vi "MyrioProject.vi"() -> ()   [LabVIEW 2018]
doc: "The myRIO Project template acquires acceleration data from the onboard accelerometer and displays the changes of acceleration values in a waveform chart."
uses:
  <vilib>/myRIO/Common/Instrument Driver Framework/Utilities/typedefs/Generic FPGA Reference.ctl
  <vilib>/myRIO/Common/Instrument Driver Framework/Utilities/typedefs/myRIO v1.0 Reference.ctl
  <vilib>/myRIO/Common/Instrument Driver Framework/Utilities/typedefs/Hardware Version Enum.ctl
  <vilib>/myRIO/Common/Instrument Driver Framework/Utilities/typedefs/myRIO Generic Hardware Reference.ctl
  <vilib>/userdefined/High Color/nirio_resource_hc.ctl
  <vilib>/myRIO/Common/Instrument Driver Framework/myRIO v1.0/Encoder/typedefs/Encoder Channels Enum.ctl
  <vilib>/myRIO/Instrument Drivers/Onboard IO/Encoder/typedefs/Encoder Reference.ctl
  <vilib>/myRIO/Instrument Drivers/Onboard IO/Encoder/Encoder.lvlib
  <vilib>/myRIO/Common/Instrument Driver Framework/myRIO v1.0/Encoder/typedefs/Encoder Signal Mode.ctl
  <vilib>/myRIO/Instrument Drivers/Onboard IO/Encoder/vis/myRIO Encoder Open.xnode
  <vilib>/myRIO/Common/Instrument Driver Framework/myRIO v1.0/Encoder/vis/myRIO v1.1 Open Encoder.vi
  <vilib>/myRIO/Common/Instrument Driver Framework/myRIO v1.0/Encoder/vis/myRIO v1.0 Configure Encoder.vi
  <vilib>/myRIO/Common/Instrument Driver Framework/myRIO v1.0/Encoder/typedefs/Encoder Configuration v1.0.ctl
  <vilib>/myRIO/Instrument Drivers/Onboard IO/PWM/typedefs/PWM Configuration.ctl
  <vilib>/myRIO/Instrument Drivers/Onboard IO/PWM/PWM.lvlib
  <vilib>/myRIO/Common/Instrument Driver Framework/myRIO v1.0/PWM/typedefs/PWM Channels Enum.ctl
  <vilib>/myRIO/Instrument Drivers/Onboard IO/PWM/typedefs/PWM Reference.ctl
  <vilib>/myRIO/Instrument Drivers/Onboard IO/PWM/vis/myRIO PWM Open.xnode
  <vilib>/myRIO/Common/Instrument Driver Framework/myRIO v1.0/PWM/vis/myRIO v1.1 Open PWM.vi
  <vilib>/myRIO/Express VI/Onboard Devices/Button/Button Express VI.xnode
  <vilib>/myRIO/Instrument Drivers/Onboard IO/DIO/typedefs/DIO Reference.ctl
  <vilib>/myRIO/Instrument Drivers/Onboard IO/DIO/DIO.lvlib
  <vilib>/myRIO/Common/Instrument Driver Framework/myRIO v1.0/DIO/typedefs/DIO Channels List.ctl
  <vilib>/myRIO/Common/Instrument Driver Framework/myRIO v1.0/DIO/typedefs/DIO Channels Enum.ctl
  <vilib>/myRIO/Instrument Drivers/Onboard IO/DIO/vis/myRIO DIO Open.xnode
  <vilib>/myRIO/Common/Instrument Driver Framework/myRIO v1.0/DIO/vis/myRIO v1.1 Open DIO.vi
  <vilib>/myRIO/Common/Instrument Driver Framework/Utilities/vis/Is FPGA Ref Available.vi
  <vilib>/myRIO/Express VI/Onboard IO/DO/DO Express VI.xnode
  <vilib>/myRIO/Instrument Drivers/Onboard IO/DIO/vis/Write.vi
  <vilib>/myRIO/Express VI/Onboard IO/AI/AI Express VI.xnode
  <vilib>/myRIO/Instrument Drivers/Onboard IO/AI/typedefs/AI Reference.ctl
  <vilib>/myRIO/Instrument Drivers/Onboard IO/AI/AI.lvlib
  <vilib>/myRIO/Common/Instrument Driver Framework/Utilities/typedefs/Analog Scaling Constants List.ctl
  <vilib>/myRIO/Common/Instrument Driver Framework/Utilities/typedefs/Analog Scaling Constants.ctl
  <vilib>/myRIO/Common/Instrument Driver Framework/myRIO v1.0/AI/typedefs/AI Channels List.ctl
  <vilib>/myRIO/Common/Instrument Driver Framework/myRIO v1.0/AI/typedefs/AI Channels Enum.ctl
  <vilib>/myRIO/Instrument Drivers/Onboard IO/AI/vis/myRIO AI Open.xnode
  <vilib>/myRIO/Common/Instrument Driver Framework/myRIO v1.0/AI/vis/myRIO v1.1 Open AI.vi
  <vilib>/myRIO/Express VI/Onboard IO/PWM/PWM Express VI.xnode
  <vilib>/myRIO/Instrument Drivers/Onboard IO/PWM/vis/Set Duty Cycle and Frequency.vi
  <vilib>/platform/TimedLoop/XDataNode/XDataNode.xnode
  <vilib>/Platform/TimedLoop/XDataNode/timing_clust.ctl
  <vilib>/Platform/TimedLoop/XDataNode/XDNodeRunTimeDep.lvlib
  <vilib>/Platform/TimedLoop/XDataNode/wakeup.ctl
  <vilib>/Platform/TimedLoop/XDataNode/nitl_modes.ctl
  <vilib>/Analysis/Matrix/Datatypes/RealMatrix.ctl
  <vilib>/Analysis/Matrix/NI_Matrix.lvlib
panel:
  in  "Garra":bool
  out "stall":bool
  in  "Start":bool
  in  "Stop Button":bool
  out "element":dbl
  out "element 2":dbl
  in  "manual":bool
  out "Numeric Control":dbl
  out "data":dbl
  out "sensor2 (A/AI2 (Pin 7))":dbl
  out "sensor1":dbl
  out "stallRojo (A/AI0 (Pin 3))":dbl
  out "stallBlanco (A/AI1 (Pin 5))":dbl
  out "subarray 2":dbl[][](array[numeric])
  out "subarray":dbl[][](array[numeric])
  out "vectores":dbl[][][](array[numeric])
  in  "saturacion":dbl=0.3
  in  "Garra":dbl(slide)=0.5 scale=0.05..0.1
  in  "Subir":dbl(slide)=0.5 scale=0.05..0.15
  in  "Reset Counter 2":bool
  in  "Reset Counter":bool
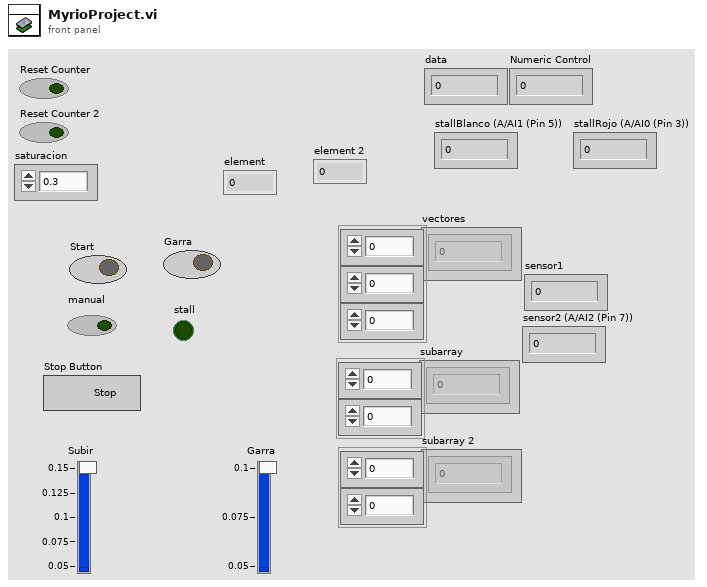
[diagram p1: front panel]
types:
  T1 = enum16{"Up-Closed", "Baja-abre", "cierra", "sube"}
  T2 = typedef "NI_Matrix.lvlib/RealMatrix.ctl" = dbl[][]
  T3 = enum16{"normal", "grande-Sensor", "grande home", "peque-sensor", "peque- home", "peque-reset"}
  T4 = typedef "Encoder Signal Mode.ctl" = enum16{"Quadrature phase signal", "Step and direction signal"}
  T5 = typedef "PWM.lvlib/PWM Reference.ctl" = cluster{"myRIO Reference":T6, "PWM Channels Enum":T10, "PWM Configuration":T11}
  T6 = typedef "myRIO Generic Hardware Reference.ctl" = cluster{"myRIO Model":T7, "myRIO Hardware Reference":T8}
  T7 = typedef "Hardware Version Enum.ctl" = enum16{"Unknown", "myRIO-1900", "myRIO-1950", "roboRIO", "NI ELVIS RIO CM", "ELVIS III"}
  T8 = typedef "myRIO v1.0 Reference.ctl" = cluster{"Generic FPGA Reference":T9, "Allow multiple opens":bool}
  T9 = typedef "Generic FPGA Reference.ctl" = refnum<k20>
  T10 = typedef "PWM Channels Enum.ctl" = enum16{"Not Connected", "C/PWM0", "C/PWM1", "A/PWM0", "A/PWM1", "A/PWM2", "A/PWM3", "A/PWM4", "A/PWM5", "A/PWM6", "A/PWM7", "A/PWM8", "A/PWM9", "A/PWM10", "A/PWM11", "A/PWM12", "A/PWM13", "A/PWM14", "A/PWM15", "A/PWM16", "A/PWM17", "A/PWM18", "A/PWM19", "B/PWM0", "B/PWM1", "B/PWM2", "B/PWM3", "B/PWM4", "B/PWM5", "B/PWM6", "B/PWM7", "B/PWM8", "B/PWM9", "B/PWM10", "B/PWM11", "B/PWM12", "B/PWM13", "B/PWM14", "B/PWM15", "B/PWM16", "B/PWM17", "B/PWM18", "B/PWM19", "PWM/PWM0", "PWM/PWM1", "PWM/PWM2", "PWM/PWM3", "PWM/PWM4", "PWM/PWM5", "PWM/PWM6", "PWM/PWM7", "PWM/PWM8", "PWM/PWM9"}
  T11 = typedef "PWM.lvlib/PWM Configuration.ctl" = cluster{"Frequency":dbl, "Duty Cycle":dbl}
  T12 = typedef "Encoder.lvlib/Encoder Reference.ctl" = cluster{"myRIO Reference":T6, "Encoder Channels Enum":T13}
  T13 = typedef "Encoder Channels Enum.ctl" = enum16{"Not Connected", "C/ENC0", "C/ENC1", "A/ENC", "A/ENC0", "A/ENC1", "A/ENC2", "A/ENC3", "A/ENC4", "A/ENC5", "A/ENC6", "A/ENC7", "A/ENC8", "A/ENC9", "B/ENC", "B/ENC0", "B/ENC1", "B/ENC2", "B/ENC3", "B/ENC4", "B/ENC5", "B/ENC6", "B/ENC7", "B/ENC8", "B/ENC9", "DIO/ENC0", "DIO/ENC1", "DIO/ENC2", "DIO/ENC3", "DIO/ENC4"}
  T14 = typedef "XDNodeRunTimeDep.lvlib/timing_clust.ctl" = cluster{"Expected End [f-1]":u64, "Actual End [f-1]":u64, "Finished Late? [f-1]":bool, "Expected End [i-1]":u64, "Actual End [i-1]":u64, "Finished Late? [i-1]":bool, "Expected Start [i]":u64, "Actual Start [i]":u64, "Expected Start [f]":u64, "Actual Start [f]":u64, "Source Name":string, "Structure Name":string, "Period":i64, "Deadline":i64, "Offset":i64, "Start":i64, "Priority":i32, "Timeout":i32, "Mode":T15, "Wakeup Reason":T16, "Error":errorcluster, "Source Type":string, "Secondary Source Type":string, "Global End Time":u64, "Global Start Time":u64, "Frame Duration":u64, "Iteration Duration":u64, "Assigned CPU":i32, "I/O Scan Engine Mode":u32}
  T15 = typedef "XDNodeRunTimeDep.lvlib/nitl_modes.ctl" = enum32{"No Change", "Process missed periods, maintain original phase", "Discard missed periods, maintain original phase", "Process missed periods, ignore original phase", "Discard missed periods, ignore original phase"}
  T16 = typedef "XDNodeRunTimeDep.lvlib/wakeup.ctl" = enum32{"Normal", "Aborted", "Asynchronous wakeup", "Timing source error", "Timed loop error", "Timeout"}
  T17 = cluster{"Double":dbl, "dbl Scaled Value":dbl, "Output":dbl, "seconds since 1Jan1904":timestamp, dbl, dbl, dbl}
  T18 = typedef "nirio_resource_hc.ctl" = tag
  T19 = typedef "AI.lvlib/AI Reference.ctl" = cluster{"myRIO Reference":T6, "AI Channels List":T20, "AI Scaling Constants List":T22}
  T20 = typedef "AI Channels List.ctl" = T21[]
  T21 = typedef "AI Channels Enum.ctl" = enum16{"Not Connected", "AudioIn/Left", "AudioIn/Right", "C/AI0", "C/AI1", "A/AI0", "A/AI1", "A/AI2", "A/AI3", "A/AI4", "A/AI5", "A/AI6", "A/AI7", "B/AI0", "B/AI1", "B/AI2", "B/AI3", "B/AI4", "B/AI5", "B/AI6", "B/AI7", "AI/AI0", "AI/AI1", "AI/AI2", "AI/AI3", "A/AI0 (DIFF)", "A/AI1 (DIFF)", "A/AI2 (DIFF)", "A/AI3 (DIFF)", "B/AI0 (DIFF)", "B/AI1 (DIFF)", "B/AI2 (DIFF)", "B/AI3 (DIFF)"}
  T22 = typedef "Analog Scaling Constants List.ctl" = T23[]
  T23 = typedef "Analog Scaling Constants.ctl" = cluster{"LSB Weight (Volts)":dbl, "Offset (Volts)":dbl, "Signed?":bool}
  T24 = typedef "DIO.lvlib/DIO Reference.ctl" = cluster{"myRIO Reference":T6, "DIO Channels List":T25}
  T25 = typedef "DIO Channels List.ctl" = T26[]
  T26 = typedef "DIO Channels Enum.ctl" = enum16{"Not Connected", "C/DIO0", "C/DIO1", "C/DIO2", "C/DIO3", "C/DIO4", "C/DIO5", "C/DIO6", "C/DIO7", "A/DIO0", "A/DIO1", "A/DIO2", "A/DIO3", "A/DIO4", "A/DIO5", "A/DIO6", "A/DIO7", "A/DIO8", "A/DIO9", "A/DIO10", "A/DIO11", "A/DIO12", "A/DIO13", "A/DIO14", "A/DIO15", "A/DIO16", "A/DIO17", "A/DIO18", "A/DIO19", "B/DIO0", "B/DIO1", "B/DIO2", "B/DIO3", "B/DIO4", "B/DIO5", "B/DIO6", "B/DIO7", "B/DIO8", "B/DIO9", "B/DIO10", "B/DIO11", "B/DIO12", "B/DIO13", "B/DIO14", "B/DIO15", "B/DIO16", "B/DIO17", "B/DIO18", "B/DIO19", "LED0", "LED1", "LED2", "LED3", "Button0", "DIO/DIO0", "DIO/DIO1", "DIO/DIO2", "DIO/DIO3", "DIO/DIO4", "DIO/DIO5", "DIO/DIO6", "DIO/DIO7", "DIO/DIO8", "DIO/DIO9", "SPI/CS0", "SPI/CS1", "SPI/CS2", "SPI/CS3", "LED RADIO (Green)", "LED RADIO (Red)", "LED COMM (Green)", "LED COMM (Red)", "LED MODE (Green)", "LED MODE (Red)"}
  T27 = cluster{dbl, dbl, "Counter Value":i32, "seconds since 1Jan1904":timestamp, dbl, dbl, "Counter Value":i32}
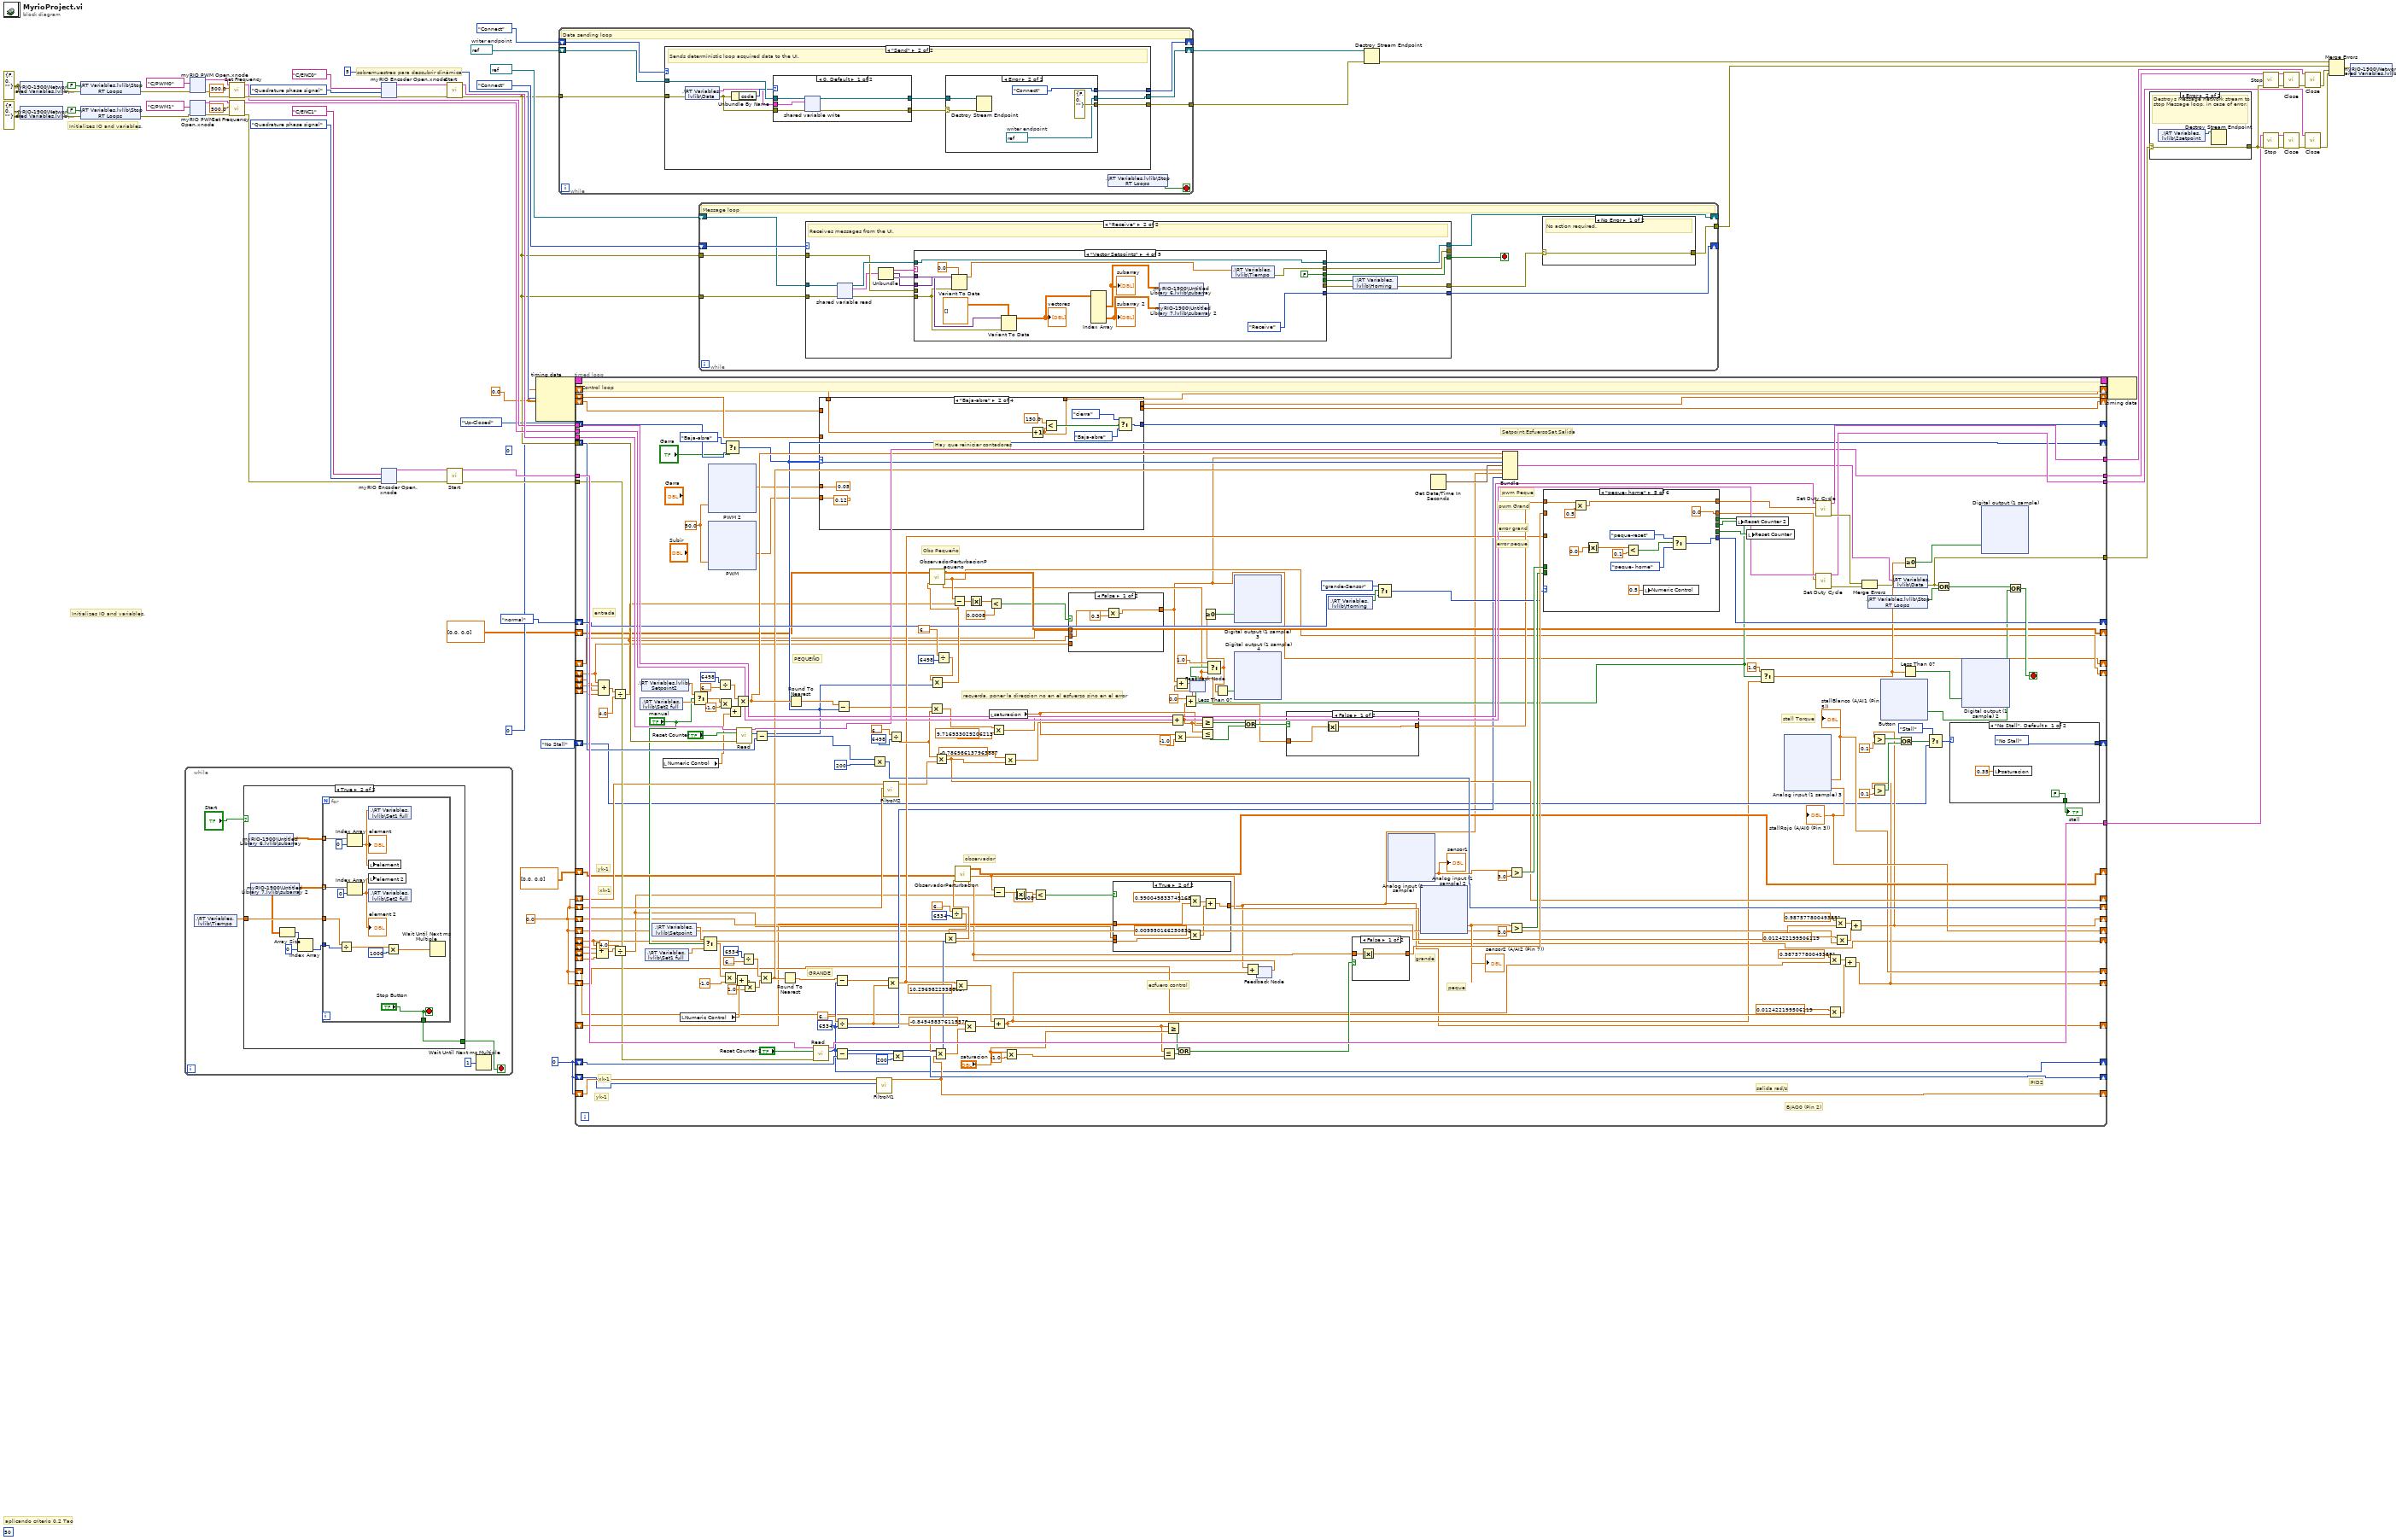
[diagram p0: block diagram]
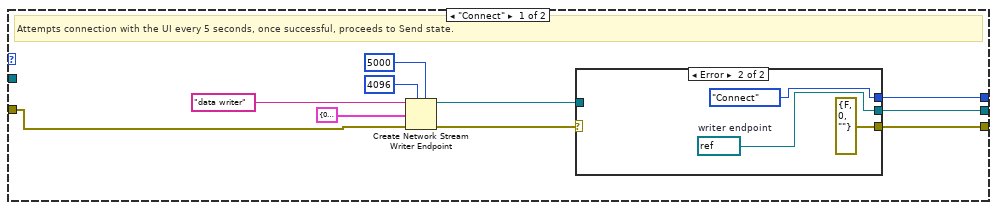
[diagram p4: hidden frame]
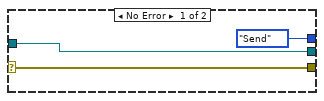
[diagram p5: hidden frame]
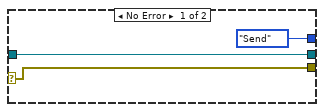
[diagram p6: hidden frame]
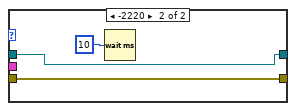
[diagram p7: hidden frame]
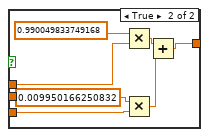
[diagram p8: hidden frame]
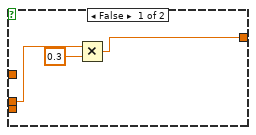
[diagram p9: hidden frame]
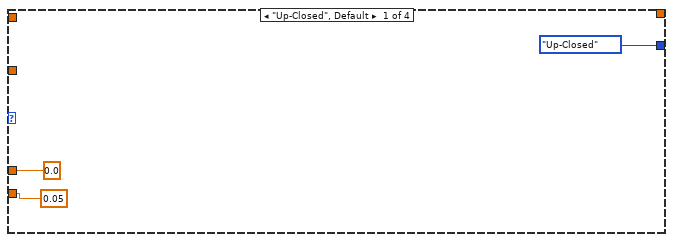
[diagram p10: hidden frame]
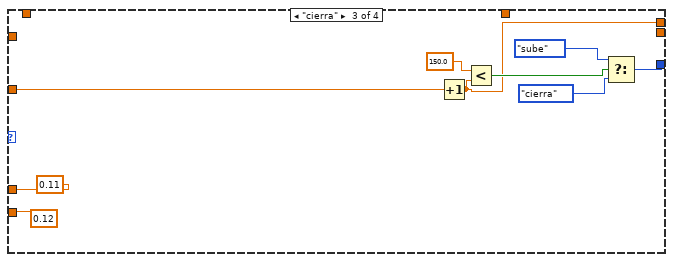
[diagram p11: hidden frame]
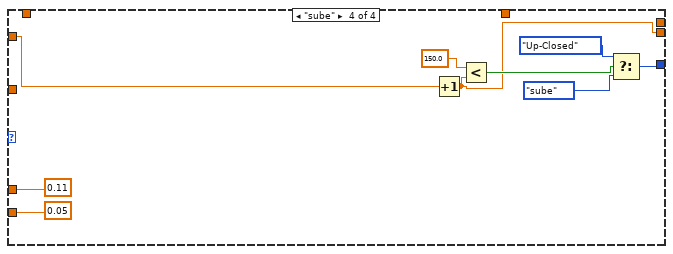
[diagram p12: hidden frame]
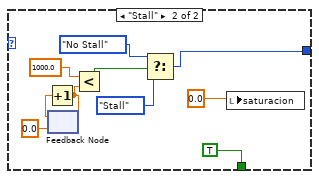
[diagram p13: hidden frame]
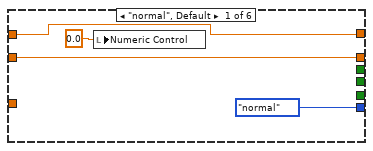
[diagram p14: hidden frame]
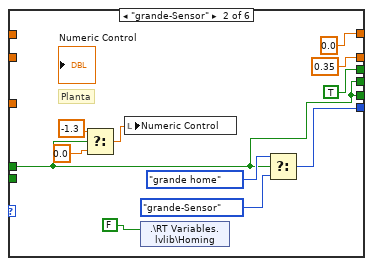
[diagram p15: hidden frame]
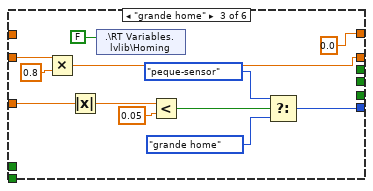
[diagram p16: hidden frame]
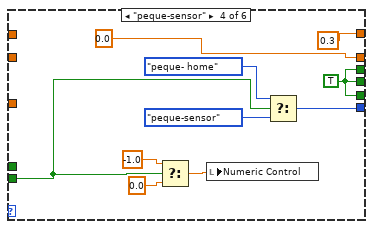
[diagram p17: hidden frame]
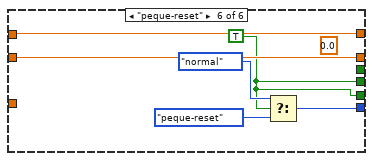
[diagram p18: hidden frame]
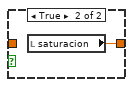
[diagram p19: hidden frame]
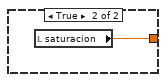
[diagram p20: hidden frame]
diagram:
  w1 = 0.0
  w4 = 0.0
  w5 = 0 ("Counter Value")
  (unwired) 0
  (unwired) 50
  w21 = refnum<k21> refnum  # writer endpoint
  w34 = errorcluster {"status"=FALSE, "code"=0, "source"=""} ("error IO")
  w56 = errorcluster {"status"=FALSE, "code"=0, "source"=""} ("error IO")
  # "aplicando criterio 0.2 Tao"
  # "sobremuestreo para descubrir dinámica"
  # "Initializes IO and variables."
  # "Initializes IO and variables."
  n1 = shared-variable "myRIO-1900\\Network Shared Variables.lvlib\\error IO"(w56, error in=w56) -> (error out=w57:errorcluster)
  n2 = shared-variable "myRIO-1900\\Network Shared Variables.lvlib\\error IO"(w34, error in=w34) -> (error out=w35:errorcluster)
  n3 = shared-variable ".\\RT Variables.lvlib\\Stop RT Loops"(FALSE ("Stop RT Loops"), error in=w57) -> (error out=w44:errorcluster)
  n4 = shared-variable ".\\RT Variables.lvlib\\Stop RT Loops"(FALSE ("Stop RT Loops"), error in=w35) -> (error out=w27:errorcluster)
  n5 = while {
    stop <- w68 stop-if-true
    n6 = shared-variable ".\\RT Variables.lvlib\\Tiempo"() -> (w70:dbl)  [unwired: 1 in, 1 out]
    n7 = case shown="True" "Start" {
      tunnel: w70 -> [_ w77]
      tunnel: [_ w76] -> w68
      frame False {
      }
      frame True {
        n8 = shared-variable "myRIO-1900\\Untitled Library 6.lvlib\\subarray"() -> (w78:dbl[][])  [unwired: 1 in, 1 out]
        n9 = shared-variable "myRIO-1900\\Untitled Library 7.lvlib\\subarray 2"() -> (w75:dbl[][])  [unwired: 1 in, 1 out]
        n10 = Array Size(array=w75) -> (size(s)=w73:i32[])
        n11 = Index Array(array=w73, index=0) -> (element=w72:i32)
        n12 = for {
          tunnel: w78 -> [w88] mode=indexing
          tunnel: w75 -> [w85] mode=indexing
          tunnel: w77 -> [w81]
          tunnel: ["Stop Button"] -> w76
          tunnel: w72 -> [w79]
          stop <- "Stop Button" stop-if-true
          n13 = Divide(x=w81, y=w79) -> (x/y=w90:dbl)
          n14 = Index Array(array=w88, index=0) -> (element=w83:dbl)
          "element" <- w83
          n15 = Index Array(array=w85, index=0) -> (element=w82:dbl)
          "element 2" <- w82
          n16 = shared-variable ".\\RT Variables.lvlib\\Set1 full"(w83) -> ()  [unwired: 1 in, 1 out]
          n17 = local write "element"(w83) -> ()
          n18 = local write "element 2"(w82) -> ()
          n19 = shared-variable ".\\RT Variables.lvlib\\Set2 full"(w82) -> ()  [unwired: 1 in, 1 out]
          n20 = Multiply(x=w90, y=1000) -> (x*y=w84:dbl)
          n21 = Wait Until Next ms Multiple(millisecond multiple=w84) -> ()  [unwired: 1 out]
        }
      }
    }
    n22 = Wait Until Next ms Multiple(millisecond multiple=u32 1) -> ()  [unwired: 1 out]
  }
  n23 = xnode "myRIO PWM Open.xnode"("error in (no error)"=w44, "Channel Name"=tag "C/PWM0") -> ("error out"=w46:errorcluster, "PWM Ref Out"=w45:T5)  [unwired: 1 in]
  n24 = xnode "myRIO PWM Open.xnode"("error in (no error)"=w27, "Channel Name"=tag "C/PWM1") -> ("error out"=w29:errorcluster, "PWM Ref Out"=w28:T5)  [unwired: 1 in]
  n25 = call <vilib>:"Set Frequency.vi"("error in (no error)"=w46, "Frequency [Hz]"=500.0, "PWM Ref In"=w45) -> ("error out"=w43:errorcluster, "PWM Ref Out"=w40:T5)  [unwired: 6 in]
  n26 = call <vilib>:"Set Frequency.vi"("error in (no error)"=w29, "Frequency [Hz]"=500.0, "PWM Ref In"=w28) -> ("error out"=w26:errorcluster, "PWM Ref Out"=w22:T5)  [unwired: 6 in]
  n27 = xnode "myRIO Encoder Open.xnode"("error in (no error)"=w43, "Channel Name"=tag "C/ENC0", "Encoder Signal Mode"=Encoder_Signal_Mode."Quadrature phase signal") -> ("error out"=w53:errorcluster, "Encoder Ref Out"=w52:T12)  [unwired: 2 in]
  n28 = xnode "myRIO Encoder Open.xnode"("error in (no error)"=w26, "Channel Name"=tag "C/ENC1", "Encoder Signal Mode"=Encoder_Signal_Mode."Quadrature phase signal") -> ("error out"=w32:errorcluster, "Encoder Ref Out"=w31:T12)  [unwired: 2 in]
  n29 = call <vilib>:"Start.vi"("error in (no error)"=w53, "Encoder Ref In"=w52) -> ("error out"=w11:errorcluster, "Encoder Ref Out"=w50:T12)  [unwired: 8 in]
  n30 = call <vilib>:"Start.vi"("error in (no error)"=w32, "Encoder Ref In"=w31) -> ("error out"=w10:errorcluster, "Encoder Ref Out"=w23:T12)  [unwired: 8 in]
  n31 = node-c288(i64 5 ("Period")) -> (w67:T14)  [unwired: 3 in]
  n32 = while {
    shift-right: [w95] -> w62
    shift-left: w21 -> [w93]
    tunnel: [w94] -> w63
    tunnel: w11 -> [w92]
    shift-right: [w91] -> _
    shift-left: enum16{"Connect", "Send"}."Connect" ("Message states") -> [w96]
    stop <- w97 stop-if-true
    # "Data sending loop"
    n33 = case shown="\"Send\"" w96 {
      tunnel: [w101 w116] -> w94
      tunnel: [w99 w114] -> w95
      tunnel: [w105 w117] -> w91
      tunnel: w93 -> [_ w123]
      tunnel: w92 -> [w102 w122]
      frame "Connect" {
        # "Attempts connection with the UI every 5 seconds, once successful, proceeds to Send state."
        n34 = Create Network Stream Writer Endpoint(5:5000 ("timeout in ms (-1)"), 7:4096 ("writer buffer size"), 8:w102, 9:T17 {"Double"=0.0, "dbl Scaled Value"=0.0, "Output"=0.0, "seconds since 1Jan1904"=timestamp(0 s since 1904-01-01), 0.0, 0.0, 0.0} ("Data"), 11:"data writer" ("writer name")) -> (0:w103:errorcluster, 3:w100:refnum<k21>)  [unwired: 2 in]
        n35 = case shown="Error" w103 {
          selector: w103 -> [w108 _]
          tunnel: [enum16{"Connect", "Send"}."Send" ("Message states") enum16{"Connect", "Send"}."Connect" ("Message states")] -> w105
          tunnel: [w108 errorcluster {"status"=FALSE, "code"=0, "source"=""} ("error IO")] -> w101
          tunnel: w100 -> [w110 _]
          tunnel: [w110 w111] -> w99
          frame No Error {
          }
          frame Error {
            w111 = refnum<k21> refnum  # writer endpoint
          }
        }
      }
      frame "Send" {
        # "Sends deterministic loop acquired data to the UI."
        n36 = shared-variable ".\\RT Variables.lvlib\\Data"(error in=w122) -> (w119:T17, error out=w121:errorcluster)
        n37 = Unbundle By Name(w121) -> ("code"=w120:i32)
        n38 = case shown="0, Default" w120 {
          tunnel: [w136 w138] -> w118
          tunnel: [w135 w137] -> w115
          tunnel: w123 -> [w134 w137]
          tunnel: w121 -> [w133 w138]
          tunnel: w119 -> [w132 _]
          frame 0, Default {
            n39 = shared-variable-write(w134, w133, w132) -> (w135:refnum<k21>, w136:errorcluster)  [unwired: 1 in, 1 out]
          }
          frame -2220 {
            n40 = Wait (ms)(milliseconds to wait=u32 10) -> ()  [unwired: 1 out]
          }
        }
        n41 = case shown="Error" w118 {
          selector: w118 -> [w126 w130]
          tunnel: [enum16{"Connect", "Send"}."Send" ("Message states") enum16{"Connect", "Send"}."Connect" ("Message states")] -> w117
          tunnel: [w126 errorcluster {"status"=FALSE, "code"=0, "source"=""} ("error IO")] -> w116
          tunnel: w115 -> [w124 w129]
          tunnel: [w124 w127] -> w114
          frame No Error {
          }
          frame Error {
            w127 = refnum<k21> refnum  # writer endpoint
            n42 = Destroy Stream Endpoint(8:w130, 11:w129) -> ()  [unwired: 1 out]
          }
        }
      }
    }
    n43 = shared-variable ".\\RT Variables.lvlib\\Stop RT Loops"() -> (w97:bool)  [unwired: 1 in, 1 out]
  }
  n44 = timed-loop {
    timing: w67 -> [_]
    timing-out: [_] -> w66
    tunnel: [w348] -> w55
    tunnel: w50 -> [w327]
    tunnel: [w326] -> w47
    tunnel: w40 -> [w317]
    tunnel: [w347] -> w39
    tunnel: w23 -> [w344]
    tunnel: w22 -> [w343]
    tunnel: [w339] -> w16
    tunnel: [w338] -> w15
    shift-right: [w316] -> _
    shift-left: T3."normal" ("Enum") -> [w315]
    shift-right: [w240] -> _
    shift-left: 0 -> [w305]
    tunnel: w10 -> [w303]
    tunnel: w11 -> [w302]
    shift-right: [w245] -> _
    shift-left: w5 -> [w260]
    shift-right: [w256] -> _
    shift-left: w5 -> [w254]
    shift-right: [w253] -> _
    shift-left: w5 -> [w255]
    shift-right: [w252] -> _
    shift-left: w4 -> [w251]
    shift-right: [w248] -> _
    shift-left: w4 -> [w250]
    shift-right: [w238] -> _
    shift-left: T2 [[0.0], [0.0]] ("A + B") -> [w239]
    shift-right: [w236] -> _
    shift-left: T2 [[0.0], [0.0]] ("A + B") -> [w235]
    shift-right: [w205] -> _
    shift-left: w4 -> [w215]
    shift-right: [w204] -> _
    shift-left: w4 -> [w210]
    shift-right: [w209] -> _
    shift-left: w4 -> [w208]
    shift-right: [w207] -> _
    shift-left: w4 -> [w206]
    shift-right: [w191] -> _
    shift-left: enum16{"No Stall", "Stall"}."No Stall" -> [w190]
    shift-right: [w186] -> _
    shift-left: T1."Up-Closed" -> [w185]
    shift-right: [w182] -> _
    shift-left: w1 -> [w183]
    shift-right: [w178] -> _
    shift-left: w1 -> [w181]
    shift-right: [w179] -> _
    shift-left: w1 -> [w180]
    shift-right: [w142] -> _
    shift-left: _ -> [w153]
    shift-right: [w159] -> _
    shift-left: _ -> [w154]
    shift-right: [w146] -> _
    shift-left: _ -> [w152]
    shift-left: _ -> [w173]
    shift-left: _ -> [w172]
    shift-left: _ -> [w171]
    shift-left: _ -> [w164]
    shift-left: _ -> [w163]
    shift-left: _ -> [w162]
    shift-right: [w143] -> _
    shift-left: _ -> [w151]
    stop <- w336 stop-if-true
    w304 = 50.0 ("Frequency [Hz]")
    # "recuerda, poner la direccion no en el esfuerzo sino en el error"
    # "entrada"
    # "error peque"
    # "error grand"
    # "pwm Grand"
    # "pwm Peque"
    # "esfuero control"
    # "Obs Pequeño"
    # "observador"
    # "yk-1"
    # "xk-1"
    # "yk-1"
    # "xk-1"
    # "PEQUEÑO"
    # "peque"
    # "grande"
    # "stall Torque"
    # "Setpoint,EsfuersoSat,Salida"
    # "PID2"
    # "GRANDE"
    # "salida rad/s"
    # "B/AO0 (Pin 2)"
    # "Control loop"
    n45 = Compound Arithmetic op=ADD(w152, w173, w172, w171) -> (w170:dbl)
    n46 = Compound Arithmetic op=ADD(w154, w164, w163, w162) -> (w161:dbl)
    n47 = Divide(x=w161, y=4.0) -> (x/y=w140:dbl)
    n48 = Divide(x=w170, y=4.0) -> (x/y=w141:dbl)
    n49 = shared-variable ".\\RT Variables.lvlib\\Set2 full"() -> (w227:dbl)  [unwired: 1 in, 1 out]
    n50 = shared-variable ".\\RT Variables.lvlib\\Setpoint2"() -> (w228:dbl)  [unwired: 1 in, 1 out]
    n51 = shared-variable ".\\RT Variables.lvlib\\Set1 full"() -> (w224:dbl)  [unwired: 1 in, 1 out]
    n52 = shared-variable ".\\RT Variables.lvlib\\Setpoint"() -> (w225:dbl)  [unwired: 1 in, 1 out]
    n53 = local read "Numeric Control"() -> (w221:dbl)
    n54 = local read "Numeric Control"() -> (w276:dbl)
    n55 = Select(t=w228, s="manual", f=w227) -> (s? t:f=w226:dbl)
    n56 = Select(t=w225, s="manual", f=w224) -> (s? t:f=w223:dbl)
    n57 = Divide(x=6498, y=6.283185307179586) -> (x/y=w297:dbl)
    n58 = Multiply(x=w226, y=-1.0) -> (x*y=w230:dbl)
    n59 = Multiply(x=w223, y=-1.0) -> (x*y=w275:dbl)
    n60 = Select(t=T1."Baja-abre", s="Garra", f=w185) -> (s? t:f=w188:T1)
    n61 = Add(x=w230, y=w221) -> (x+y=w229:dbl)
    n62 = Add(x=w275, y=w276) -> (x+y=w233:dbl)
    n63 = Multiply(x=w297, y=w229) -> (x*y=w272:dbl)
    n64 = call <vilib>:"Read.vi"("error in (no error)"=w302, "Reset Counter"="Reset Counter", "Encoder Ref In"=w327) -> ("Counter Value"=w240:i32, "Encoder Ref Out"=w326:T12)  [unwired: 4 in, 3 out]
    n65 = Divide(x=6534, y=6.283185307179586) -> (x/y=w294:dbl)
    n66 = Multiply(x=w233, y=1.0) -> (x*y=w231:dbl)
    n67 = Subtract(x=w240, y=w305) -> (x-y=w283:i32)
    n68 = Multiply(x=w294, y=w231) -> (x*y=w268:dbl)
    n69 = Round To Nearest(number=w268) -> (nearest integer value=w330:dbl)
    n70 = Round To Nearest(number=w272) -> (nearest integer value=w325:dbl)
    n71 = call <vilib>:"Read.vi"("error in (no error)"=w303, "Reset Counter"="Reset Counter 2", "Encoder Ref In"=w344) -> ("Counter Value"=w245:i32, "Encoder Ref Out"=w339:T12)  [unwired: 4 in, 3 out]
    n72 = case shown="\"Baja-abre\"" w188 {
      tunnel: [T1."Up-Closed" w380 w389 w398] -> w186
      tunnel: [0.0 0.05 0.11 0.11] -> w177
      tunnel: [0.05 0.12 0.12 0.05] -> w176
      tunnel: w183 -> [_ _ w384 _]
      tunnel: [_ _ w383 _] -> w182
      tunnel: w181 -> [_ _ _ w394]
      tunnel: w180 -> [_ w376 _ _]
      tunnel: [_ w375 _ _] -> w179
      tunnel: [_ _ _ w393] -> w178
      frame "Up-Closed", Default {
      }
      frame "Baja-abre" {
        # "Hay que reiniciar contadores"
        n73 = Increment(x=w376) -> (x+1=w375:dbl)
        n74 = Less?(x=150.0, y=w375) -> (x < y?=w377:bool)
        n75 = Select(t=T1."cierra", s=w377, f=T1."Baja-abre") -> (s? t:f=w380:T1)
      }
      frame "cierra" {
        n76 = Increment(x=w384) -> (x+1=w383:dbl)
        n77 = Less?(x=150.0, y=w383) -> (x < y?=w387:bool)
        n78 = Select(t=T1."sube", s=w387, f=T1."cierra") -> (s? t:f=w389:T1)
      }
      frame "sube" {
        n79 = Increment(x=w394) -> (x+1=w393:dbl)
        n80 = Less?(x=150.0, y=w393) -> (x < y?=w395:bool)
        n81 = Select(t=T1."Up-Closed", s=w395, f=T1."sube") -> (s? t:f=w398:T1)
      }
    }
    n82 = xnode "PWM 2"("Duty Cycle"=w177, "Frequency [Hz]"=w304) -> ()  [unwired: 1 in, 1 out]
    n83 = xnode "PWM"("Duty Cycle"=w176, "Frequency [Hz]"=w304) -> ()  [unwired: 1 in, 1 out]
    n84 = Subtract(x=w330, y=w245) -> (x-y=w220:dbl)
    n85 = Subtract(x=w245, y=w260) -> (x-y=w262:i32)
    n86 = Divide(x=6.283185307179586, y=6534) -> (x/y=w259:dbl)
    n87 = Subtract(x=w325, y=w240) -> (x-y=w203:dbl)
    n88 = Multiply(x=w283, y=200) -> (x*y=w252:i32)
    n89 = call "FiltroM1.vi"("Numeric 3"=w254, "Numeric in"=w255) -> ("Numeric out"=w253:dbl)  [unwired: 9 in]
    n90 = call "FiltroM2.vi"("entrada"=w251, "salida"=w250) -> ("Numeric out"=w249:dbl)  [unwired: 9 in]
    n91 = Multiply(x=w220, y=w259) -> (x*y=w265:dbl)
    n92 = Divide(x=6.283185307179586, y=6498) -> (x/y=w273:dbl)
    n93 = Multiply(x=w262, y=200) -> (x*y=w256:i32)
    n94 = Multiply(x=w203, y=w273) -> (x*y=w198:dbl)
    n95 = Multiply(x=w259, y=w253) -> (x*y=w261:dbl)
    n96 = Multiply(x=w273, y=w249) -> (x*y=w248:dbl)
    n97 = Divide(x=6.283185307179586, y=6498) -> (x/y=w241:dbl)
    n98 = Multiply(x=w241, y=w240) -> (x*y=w234:dbl)
    n99 = Divide(x=6.283185307179586, y=6534) -> (x/y=w244:dbl)
    n100 = Multiply(x=w244, y=w245) -> (x*y=w237:dbl)
    n101 = Multiply(x=w265, y=10.29698229388027) -> (x*y=w266:dbl)
    n102 = Multiply(x=-0.849458376115575, y=w261) -> (x*y=w258:dbl)
    n103 = local read "saturacion"() -> (w289:dbl)
    n104 = Multiply(x=w198, y=9.716933029206213) -> (x*y=w306:dbl)
    n105 = Add(x=w266, y=w258) -> (x+y=w147:dbl)
    n106 = Multiply(x=-0.786986137963887, y=w248) -> (x*y=w269:dbl)
    n107 = Multiply(x="saturacion", y=-1.0) -> (x*y=w288:dbl)
    n108 = Less Or Equal?(x=w147, y=w288) -> (x <= y?=w332:bool)
    n109 = Greater Or Equal?(x=w147, y="saturacion") -> (x >= y?=w333:bool)
    n110 = Add(x=w306, y=w269) -> (x+y=w175:dbl)
    n111 = Multiply(x=w289, y=-1.0) -> (x*y=w291:dbl)
    n112 = Or(x=w333, y=w332) -> (x .or. y?=w331:bool)
    n113 = Add(x=0.0, y=w175) -> (x+y=w150:dbl)
    n114 = feedback #1() -> (w148:dbl)  [unwired: 1 in]
    n115 = call "ObservadorPerturbacionPequeno.vi"("entrada planta"=w148, "salida planta"=w234, "xk +1"=w235) -> ("Perturbacion"=w159:dbl, "xk"=w236:T2)  [unwired: 7 in]
    n116 = Subtract(x=w159, y=w140) -> (x-y=w158:dbl)
    n117 = Absolute Value(x=w158) -> (abs(x)=w157:dbl)
    n118 = Less?(x=w157, y=0.0008) -> (x < y?=w155:bool)
    n119 = case shown="False" w155 {
      tunnel: w154 -> [_ w355]
      tunnel: w153 -> [_ w358]
      tunnel: [w353 w354] -> w142
      tunnel: w140 -> [w351 _]
      frame False {
        n120 = Multiply(x=w351, y=0.3) -> (x*y=w353:dbl)
      }
      frame True {
        n121 = Multiply(x=0.990049833749168, y=w358) -> (x*y=w356:dbl)
        n122 = Multiply(x=0.009950166250832, y=w355) -> (x*y=w357:dbl)
        n123 = Add(x=w356, y=w357) -> (x+y=w354:dbl)
      }
    }
    n124 = Add(x=w142, y=w150) -> (x+y=w149:dbl)
    n125 = feedback-in #1(w149) -> ()
    n126 = Greater Or Equal?(x=w175, y=w289) -> (x >= y?=w335:bool)
    n127 = Less Or Equal?(x=w175, y=w291) -> (x <= y?=w334:bool)
    n128 = Or(x=w335, y=w334) -> (x .or. y?=w280:bool)
    n129 = feedback #2() -> (w144:dbl)  [unwired: 1 in]
    n130 = call "ObservadorPerturbacion.vi"("entrada planta"=w144, "salida planta"=w237, "xk +1"=w239) -> ("Perturbacion"=w146:dbl, "xk"=w238:T2)  [unwired: 7 in]
    n131 = Subtract(x=w146, y=w141) -> (x-y=w168:dbl)
    n132 = Absolute Value(x=w168) -> (abs(x)=w167:dbl)
    n133 = Less?(x=w167, y=0.0008) -> (x < y?=w166:bool)
    n134 = case shown="True" w166 {
      tunnel: [w363 w365] -> w143
      tunnel: w152 -> [_ w366]
      tunnel: w151 -> [_ w364]
      tunnel: w141 -> [w361 _]
      frame False {
        n135 = Multiply(x=w361, y=0.3) -> (x*y=w363:dbl)
      }
      frame True {
        n136 = Multiply(x=0.990049833749168, y=w364) -> (x*y=w367:dbl)
        n137 = Multiply(x=0.009950166250832, y=w366) -> (x*y=w368:dbl)
        n138 = Add(x=w367, y=w368) -> (x+y=w365:dbl)
      }
    }
    n139 = Add(x=w143, y=w147) -> (x+y=w145:dbl)
    n140 = feedback-in #2(w145) -> ()
    n141 = case shown="False" w280 {
      tunnel: [w795 w796] -> w271
      tunnel: w148 -> [w794 _]
      frame False {
        n142 = Absolute Value(x=w794) -> (abs(x)=w795:dbl)
      }
      frame True {
        n143 = local read "saturacion"() -> (w796:dbl)
      }
    }
    n144 = shared-variable ".\\RT Variables.lvlib\\Homing"() -> (w318:bool)  [unwired: 1 in, 1 out]
    n145 = case shown="False" w331 {
      tunnel: [w791 w793] -> w313
      tunnel: w144 -> [w792 _]
      frame False {
        n146 = Absolute Value(x=w792) -> (abs(x)=w791:dbl)
      }
      frame True {
        n147 = local read "saturacion"() -> (w793:dbl)
      }
    }
    n148 = Select(t=T3."grande-Sensor" ("Enum"), s=w318, f=w315) -> (s? t:f=w278:T3)
    n149 = xnode "Analog input (1 sample)"() -> ("A/AI3 (Pin 9)"=w301:dbl)  [unwired: 1 in, 1 out]
    "sensor1" <- w301
    n150 = xnode "Analog input (1 sample) 2"() -> ("sensor2 (A/AI2 (Pin 7))"=w300:dbl)  [unwired: 1 in, 1 out]
    "sensor2 (A/AI2 (Pin 7))" <- w300
    n151 = Get Date/Time In Seconds() -> (seconds since 1Jan1904=w350:timestamp)
    n152 = Bundle(w272, w142, "Counter Value"=w240, "seconds since 1Jan1904"=w350, w268, w143, "Counter Value"=w245) -> (w270:T27)  [unwired: 1 in]
    n153 = Greater?(x=w301, y=3.0) -> (0:w314:bool)
    n154 = Greater?(x=w300, y=3.0) -> (0:w312:bool)
    n155 = case shown="\"peque- home\"" w278 {
      tunnel: w271 -> [w484 _ _ _ w524 w535]
      tunnel: [T3."normal" ("Enum") w498 w510 w520 w532 w537] -> w316
      tunnel: w314 -> [_ w493 _ _ _ _]
      tunnel: w313 -> [w487 _ w501 _ _ w534]
      tunnel: [w487 0.35 ("f") w499 0.0 ("f") 0.0 ("f") w534] -> w194
      tunnel: w312 -> [_ _ _ w512 _ _]
      tunnel: [w484 0.0 ("f") 0.0 0.3 ("f") w522 w535] -> w195
      tunnel: [_ w493 _ w516 _ w533] -> w310
      tunnel: [_ w493 _ w516 _ w533] -> w308
      tunnel: [_ TRUE _ w516 _ _] -> w201
      tunnel: w265 -> [_ _ w507 _ _ _]
      frame "normal", Default {
        n156 = local write "Numeric Control"(0.0) -> ()
      }
      frame "grande-Sensor" {
        # "Planta"
        n157 = Select(t=-1.3, s=w493, f=0.0) -> (s? t:f=w490:dbl)
        n158 = local write "Numeric Control"(w490) -> ()
        n159 = shared-variable ".\\RT Variables.lvlib\\Homing"(FALSE) -> ()  [unwired: 1 in, 1 out]
        n160 = Select(t=T3."grande home" ("Enum"), s=w493, f=T3."grande-Sensor" ("Enum")) -> (s? t:f=w498:T3)
      }
      frame "grande home" {
        n161 = Multiply(x=w501, y=0.8) -> (x*y=w499:dbl)
        n162 = Absolute Value(x=w507) -> (abs(x)=w506:dbl)
        n163 = shared-variable ".\\RT Variables.lvlib\\Homing"(FALSE ("Homing")) -> ()  [unwired: 1 in, 1 out]
        n164 = Less?(x=w506, y=0.05) -> (x < y?=w504:bool)
        n165 = Select(t=T3."peque-sensor" ("Enum"), s=w504, f=T3."grande home" ("Enum")) -> (s? t:f=w510:T3)
      }
      frame "peque-sensor" {
        w516 = TRUE
        n166 = Select(t=-1.0, s=w512, f=0.0) -> (s? t:f=w513:dbl)
        n167 = local write "Numeric Control"(w513) -> ()
        n168 = Select(t=T3."peque- home" ("Enum"), s=w512, f=T3."peque-sensor" ("Enum")) -> (s? t:f=w520:T3)
      }
      frame "peque- home" {
        n169 = Multiply(x=w524, y=0.5) -> (x*y=w522:dbl)
        n170 = Absolute Value(x=0.0) -> (abs(x)=w529:dbl)
        n171 = Less?(x=w529, y=0.1) -> (x < y?=w527:bool)
        n172 = local write "Numeric Control"(0.5 ("Numeric Control")) -> ()
        n173 = Select(t=T3."peque-reset" ("Enum"), s=w527, f=T3."peque- home" ("Enum")) -> (s? t:f=w532:T3)
      }
      frame "peque-reset" {
        w533 = TRUE
        (unwired) 0.0 ("f")
        n174 = Select(t=T3."normal" ("Enum"), s=w533, f=T3."peque-reset" ("Enum")) -> (s? t:f=w537:T3)
      }
    }
    n175 = Select(t=1.0, s=w201, f=w148) -> (s? t:f=w202:dbl)
    n176 = Greater Or Equal To 0?(x=w202) -> (x >= 0?=w293:bool)
    n177 = Less Than 0?(x=w202) -> (x < 0?=w292:bool)
    n178 = xnode "Digital output (1 sample) 3"("A/DIO2 (Pin 15)"=w293) -> ()  [unwired: 1 in, 1 out]
    n179 = xnode "Digital output (1 sample) 4"("A/DIO3 (Pin 17)"=w292) -> ()  [unwired: 1 in, 1 out]
    n180 = local write "Reset Counter 2"(w308) -> ()
    n181 = local write "Reset Counter"(w310) -> ()
    n182 = Select(t=1.0, s=w201, f=w147) -> (s? t:f=w277:dbl)
    n183 = xnode "Analog input (1 sample) 3"() -> ("stallBlanco (A/AI1 (Pin 5))"=w207:dbl, "stallRojo (A/AI0 (Pin 3))"=w209:dbl)  [unwired: 1 in, 1 out]
    "stallBlanco (A/AI1 (Pin 5))" <- w207
    "stallRojo (A/AI0 (Pin 3))" <- w209
    n184 = call <vilib>:"Set Duty Cycle.vi"("Duty Cycle"=w195, "PWM Ref In"=w317) -> ("error out"=w341:errorcluster, "PWM Ref Out"=w347:T5)  [unwired: 7 in]
    n185 = call <vilib>:"Set Duty Cycle.vi"("Duty Cycle"=w194, "PWM Ref In"=w343) -> ("error out"=w342:errorcluster, "PWM Ref Out"=w338:T5)  [unwired: 7 in]
    n186 = Multiply(x=0.987577800493881, y=w210) -> (x*y=w212:dbl)
    n187 = Multiply(x=0.012422199506119, y=w206) -> (x*y=w211:dbl)
    n188 = Multiply(x=0.987577800493881, y=w215) -> (x*y=w217:dbl)
    n189 = Multiply(x=0.012422199506119, y=w208) -> (x*y=w216:dbl)
    n190 = Add(x=w212, y=w211) -> (x+y=w204:dbl)
    n191 = Add(x=w217, y=w216) -> (x+y=w205:dbl)
    n192 = Merge Errors(w341, w342) -> (w340:errorcluster)
    n193 = shared-variable ".\\RT Variables.lvlib\\Stop RT Loops"() -> (w349:bool)  [unwired: 1 in, 1 out]
    n194 = Greater?(x=w205, y=0.1) -> (0:w320:bool)
    n195 = Greater?(x=w204, y=0.1) -> (0:w319:bool)
    n196 = xnode "Button"() -> ("Value"=w197:bool)  [unwired: 1 in, 1 out]
    n197 = shared-variable ".\\RT Variables.lvlib\\Data"(w270, error in=w340) -> (error out=w348:errorcluster)
    n198 = Or(x=w320, y=w319) -> (x .or. y?=w196:bool)
    n199 = Greater Or Equal To 0?(x=w277) -> (x >= 0?=w285:bool)
    n200 = Less Than 0?(x=w277) -> (x < 0?=w284:bool)
    n201 = Select(t=enum16{"No Stall", "Stall"}."Stall", s=w196, f=w190) -> (s? t:f=w193:enum16{"No Stall", "Stall"})
    n202 = Or(x=w348, y=w349) -> (x .or. y?=w337:bool)
    n203 = case shown="\"No Stall\", Default" w193 {
      tunnel: [enum16{"No Stall", "Stall"}."No Stall" w406] -> w191
      tunnel: [FALSE ("stall") TRUE ("stall")] -> w189
      frame "No Stall", Default {
        n204 = local write "saturacion"(0.35 ("saturacion")) -> ()
      }
      frame "Stall" {
        n205 = feedback #3(0.0) -> (w413:dbl)
        n206 = Increment(x=w413) -> (x+1=w411:dbl)
        n207 = feedback-in #3(w411) -> ()
        n208 = Less?(x=1000.0, y=w411) -> (x < y?=w412:bool)
        n209 = Select(t=enum16{"No Stall", "Stall"}."No Stall", s=w412, f=enum16{"No Stall", "Stall"}."Stall") -> (s? t:f=w406:enum16{"No Stall", "Stall"})
        n210 = local write "saturacion"(0.0) -> ()
      }
    }
    "stall" <- w189
    n211 = xnode "Digital output (1 sample) 2"("A/DIO1 (Pin 13)"=w284) -> ()  [unwired: 1 in, 1 out]
    n212 = xnode "Digital output (1 sample)"("A/DIO0 (Pin 11)"=w285) -> ()  [unwired: 1 in, 1 out]
    n213 = Or(x=w337, y=w197) -> (x .or. y?=w336:bool)
  }
  n214 = while {
    tunnel: [w837] -> w59
    shift-right: [w841] -> _
    shift-left: refnum<k21> refnum ("reader endpoint") -> [w839]
    shift-right: [w840] -> _
    shift-left: enum16{"Connect", "Receive"}."Connect" ("Message states") -> [w842]
    tunnel: w11 -> [w838]
    tunnel: w11 -> [w835]
    stop <- w836 stop-if-true
    # "Message loop"
    n215 = case shown="\"Receive\"" w842 {
      tunnel: [w849 w866] -> _
      tunnel: [w847 w878] -> w841
      tunnel: [w856 w875] -> w840
      tunnel: w839 -> [_ w874]
      tunnel: w838 -> [_ w877]
      tunnel: [FALSE ("Stop RT Loops") w876] -> w836
      tunnel: w835 -> [_ w871]
      tunnel: [_ w867] -> w834
      frame "Connect" {
        # "Attempts connection with the UI every 5 seconds, once successful, proceeds to Receive state."
        n216 = Bundle("", variant, variant) -> (w852:cluster{string, variant, variant})  [unwired: 1 in]
        n217 = Create Network Stream Reader Endpoint(5:5000 ("timeout in ms (-1)"), 7:4096 ("reader buffer size"), 9:w852, 11:"message reader" ("reader name")) -> (0:w851:errorcluster, 3:w846:refnum<k21>)  [unwired: 3 in]
        n218 = case shown="Error" w851 {
          selector: w851 -> [w861 _]
          tunnel: [enum16{"Connect", "Receive"}."Receive" ("Message states") enum16{"Connect", "Receive"}."Connect" ("Message states")] -> w856
          tunnel: [w860 errorcluster {"status"=FALSE, "code"=0, "source"=""} ("error IO")] -> w849
          tunnel: [w859 refnum<k21> refnum ("reader endpoint")] -> w847
          tunnel: w846 -> [w859 _]
          frame No Error {
            n219 = shared-variable ".\\RT Variables.lvlib\\2setpoint"(w859, error in=w861) -> (error out=w860:errorcluster)
          }
          frame Error {
          }
        }
      }
      frame "Receive" {
        # "Receives messages from the UI."
        n220 = shared-variable-read(w874, w877) -> (w873:refnum<k21>, w879:errorcluster, w870:cluster{string, variant, variant})  [unwired: 1 in, 1 out]
        n221 = Unbundle(w870) -> (w881:string, w880:variant, w872:variant)
        n222 = case shown="\"Vector Setpoints\"" w881 {
          tunnel: w880 -> [_ w902 w917 w923 w941]
          tunnel: w879 -> [w886 w904 w906 w922 w935]
          tunnel: [w885 w899 w913 w924 _] -> w866
          tunnel: [refnum<k21> refnum ("reader endpoint") refnum<k21> refnum ("reader endpoint") w912 w930 w939] -> w878
          tunnel: w873 -> [w884 w898 w912 w930 w939]
          tunnel: [w882 w901 FALSE ("Stop RT Loops") FALSE ("Stop RT Loops") FALSE ("Stop RT Loops")] -> w876
          tunnel: [enum16{"Connect", "Receive"}."Connect" ("Message states") enum16{"Connect", "Receive"}."Receive" ("Message states") enum16{"Connect", "Receive"}."Receive" ("Message states") enum16{"Connect", "Receive"}."Receive" ("Message states") enum16{"Connect", "Receive"}."Receive" ("Message states")] -> w875
          tunnel: w872 -> [_ w894 w905 w926 w934]
          tunnel: w871 -> [_ w893 _ _ _]
          tunnel: [w882 _ _ _ w932] -> w869
          tunnel: [_ _ _ _ w931] -> w868
          frame "Disconnect UI", Default {
            w882 = FALSE ("Stop RT Loops")
            n223 = Destroy Stream Endpoint(8:w886, 11:w884) -> (0:w885:errorcluster)
          }
          frame "Stop" {
            n224 = Variant To Data(error in=w904, type=TRUE ("Stop RT Loops"), Variant=w902) -> (data=w901:bool, error out=w903:errorcluster)
            n225 = Variant To Data(error in=w893, type=TRUE ("Stop RT Loops"), Variant=w894) -> (data=w891:bool, error out=w895:errorcluster)
            n226 = shared-variable ".\\RT Variables.lvlib\\Stop RT Loops"(w901, error in=w903) -> (error out=w889:errorcluster)
            n227 = shared-variable ".\\RT Variables.lvlib\\Stop RT Loops"(w891, error in=w895) -> (error out=w890:errorcluster)
            n228 = Merge Errors(w889, w890) -> (w888:errorcluster)
            n229 = Destroy Stream Endpoint(8:w888, 11:w898) -> (0:w899:errorcluster)
          }
          frame "Update setpoint" {
            n230 = Variant To Data(error in=w906, type=0.0, Variant=w917) -> (data=w915:dbl, error out=w914:errorcluster)
            n231 = Variant To Data(error in=w906, type=0.0, Variant=w905) -> (data=w908:dbl, error out=w907:errorcluster)
            n232 = shared-variable ".\\RT Variables.lvlib\\Setpoint2"(w908, error in=w907) -> ()  [unwired: 1 out]
            n233 = shared-variable ".\\RT Variables.lvlib\\Setpoint"(w915, error in=w914) -> (error out=w913:errorcluster)
          }
          frame "Vector Setpoints" {
            n234 = Variant To Data(error in=w922, type=0.0, Variant=w926) -> (data=w925:dbl)  [unwired: 1 out]
            n235 = Variant To Data(error in=w922, type=dbl[][][] [], Variant=w923) -> (data=w920:dbl[][][])  [unwired: 1 out]
            "vectores" <- w920
            n236 = Index Array(array=w920) -> (element #1=w919:dbl[][], element #2=w918:dbl[][])  [unwired: 6 in]
            "subarray" <- w919
            "subarray 2" <- w918
            n237 = shared-variable "myRIO-1900\\Untitled Library 6.lvlib\\subarray"(w919) -> ()  [unwired: 1 in, 1 out]
            n238 = shared-variable "myRIO-1900\\Untitled Library 7.lvlib\\subarray 2"(w918) -> ()  [unwired: 1 in, 1 out]
            n239 = shared-variable ".\\RT Variables.lvlib\\Tiempo"(w925) -> (error out=w924:errorcluster)  [unwired: 1 in]
          }
          frame "Homing" {
            n240 = Variant To Data(error in=w935, type=0.0, Variant=w934) -> (data=→"data":dbl)  [unwired: 1 out]
            n241 = Variant To Data(error in=w935, type=TRUE, Variant=w941) -> (data=w932:bool, error out=w931:errorcluster)
          }
        }
        n242 = shared-variable ".\\RT Variables.lvlib\\Homing"(w869, error in=w868) -> (error out=w867:errorcluster)
      }
    }
    n243 = case shown="No Error" w834 {
      selector: w834 -> [w843 w844]
      tunnel: [w843 w844] -> w837
      frame No Error {
        # "No action required."
      }
      frame Error {
        # "Stops RT in case of error."
        n244 = shared-variable ".\\RT Variables.lvlib\\Stop RT Loops"(TRUE ("Stop RT Loops")) -> ()  [unwired: 1 in, 1 out]
      }
    }
  }
  n245 = Destroy Stream Endpoint(8:w63, 11:w62) -> (0:w60:errorcluster)
  n246 = node-c288(w66) -> ()  [unwired: 1 out]
  n247 = case shown="Error" w55 {
    selector: w55 -> [w942 w943]
    tunnel: [w942 w943] -> w17
    frame No Error {
      # "No action required."
    }
    frame Error {
      # "Destroys Message network stream to stop Message loop, in case of error."
      n248 = shared-variable ".\\RT Variables.lvlib\\2setpoint"() -> (w944:refnum<k21>)  [unwired: 1 in, 1 out]
      n249 = Destroy Stream Endpoint(11:w944) -> ()  [unwired: 1 in, 1 out]
    }
  }
  n250 = call <vilib>:"Stop.vi"("error in (no error)"=w17, "Encoder Ref In"=w47) -> ("error out"=w48:errorcluster, "Encoder Ref Out"=w49:T12)  [unwired: 8 in]
  n251 = call <vilib>:"Stop.vi"("error in (no error)"=w17, "Encoder Ref In"=w16) -> ("error out"=w19:errorcluster, "Encoder Ref Out"=w20:T12)  [unwired: 8 in]
  n252 = call <vilib>:"Close.vi"("error in (no error)"=w48, "Encoder Ref In"=w49) -> ("error out"=w42:errorcluster)  [unwired: 9 in]
  n253 = call <vilib>:"Close.vi"("error in (no error)"=w19, "Encoder Ref In"=w20) -> ("error out"=w18:errorcluster)  [unwired: 9 in]
  n254 = call <vilib>:"Close.vi"("error in (no error)"=w42, "PWM Ref In"=w39) -> ("error out"=w41:errorcluster)  [unwired: 9 in]
  n255 = call <vilib>:"Close.vi"("error in (no error)"=w18, "PWM Ref In"=w15) -> ("error out"=w14:errorcluster)  [unwired: 9 in]
  n256 = Merge Errors(w60, w59, w41, w14) -> (w58:errorcluster)
  n257 = shared-variable "myRIO-1900\\Network Shared Variables.lvlib\\error IO"(w58) -> ()  [unwired: 1 in, 1 out]
